vi "trash_Handle Late Iterations.vi"(8 "error in (no error)":errorcluster, 10 "Period (ns)":i64, 11 "CIFCorePlugin in":refnum<class "CIFCorePlugin.lvclass">) -> (0 "error out":errorcluster, 3 "CIFCorePlugin out":refnum<class "CIFCorePlugin.lvclass">)   [LabVIEW 2021, in "CIFCorePlugin.lvclass"]
uses:
  CIFCorePlugin.lvclass
  CIFCorePlugin.lvclass/CIFCorePlugin.ctl
  CIFUtilities/CIFClocks/Typedef/Errors.ctl
  Accessors/Read Iterations.vi
  Accessors/Get Time.vi
  Accessors/Timestamps/Read Running TS.vi
  CIFUtilities/CIFClocks/Core/Get Time.vi
  CIFUtilities/CIFClocks/Time Conversion/LabVIEW Time to UTC Time.vi
  CIFCoreCommon/CIFCoreCommon.lvlib
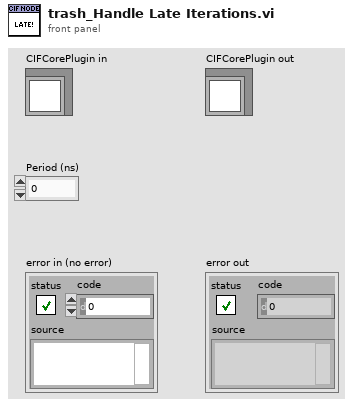
[diagram p1: front panel]
types:
  T1 = typedef "CIFCoreCommon.lvlib/Errors.ctl" = enum16{"Invalid Clock ID", "Long Sleep", "gRPC Server Not Found", "Config Parse", "Timestamp Wrap", "Delayed Execution"}
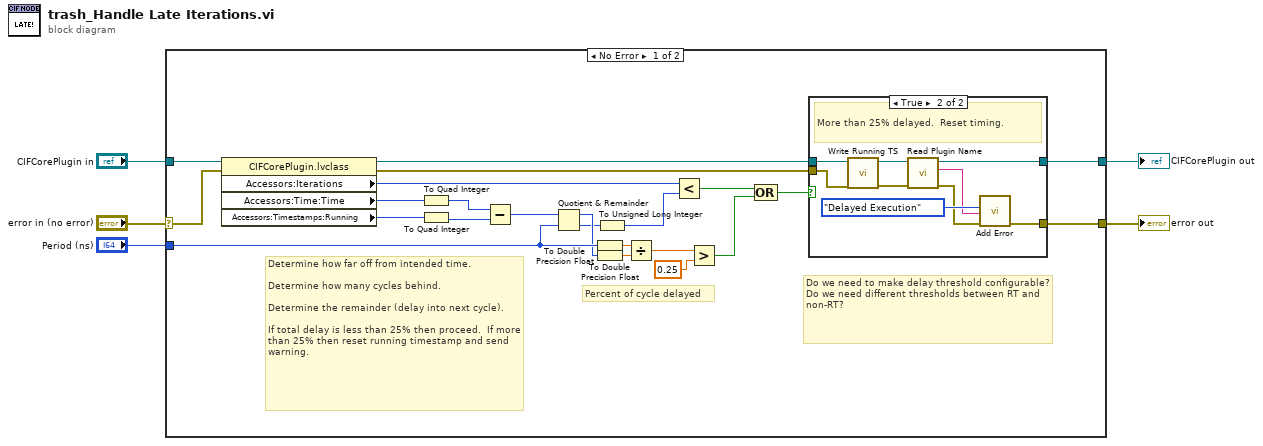
[diagram p0: block diagram]
diagram:
  n1 = case shown="No Error" "error in (no error)" {
    selector: "error in (no error)" -> [w8 w41]
    tunnel: [w7 w41] -> w4
    tunnel: [w10 w40] -> w2
    tunnel: "CIFCorePlugin in" -> [w28 w40]
    tunnel: "Period (ns)" -> [w22 _]
    frame No Error {
      # "Do we need to make delay threshold configurable?  Do we need different thresholds between RT and non-RT?"
      # "Determine how far off from intended time.\n\nDetermine how many cycles behind.\n\nDetermine the remainder (delay into next cycle).\n\nIf total delay is less than 25% then proceed.  If more than 25% then reset running timestamp and send warning."
      # "Percent of cycle delayed"
      n2 = property class="CIFCorePlugin.lvclass"(reference=w28, error in=w8) -> (reference out=w12:refnum<class "CIFCorePlugin.lvclass">, error out=w9:errorcluster, "Accessors:Iterations"=w15:u32, "Accessors:Time:Time"=w23:u64, "Accessors:Timestamps:Running"=w27:u64)
      n3 = To Quad Integer(1:w23) -> (0:w26:i64)
      n4 = To Quad Integer(1:w27) -> (0:w25:i64)
      n5 = Subtract(x=w26, y=w25) -> (x-y=w24:i64)
      n6 = Quotient & Remainder(x=w24, y=w22) -> (x-y*floor(x/y)=w21:i64, floor(x/y)=w16:i64)
      n7 = To Double Precision Float(number=w22) -> (double precision float=w19:dbl)
      n8 = To Double Precision Float(number=w21) -> (double precision float=w20:dbl)
      n9 = To Unsigned Long Integer(number=w16) -> (unsigned 32bit integer=w6:u32)
      n10 = Divide(x=w19, y=w20) -> (x/y=w18:dbl)
      n11 = Less?(x=w15, y=w6) -> (x < y?=w13:bool)
      n12 = Greater?(x=w18, y=0.25) -> (0:w14:bool)
      n13 = Compound Arithmetic op=OR(w13, w14) -> (w11:bool)
      n14 = case shown="True" w11 {
        tunnel: w12 -> [w30 w39]
        tunnel: [w30 w34] -> w10
        tunnel: w9 -> [w29 w38]
        tunnel: [w29 w33] -> w7
        frame False {
          # "Less and 25% of cycle delayed, keep running"
        }
        frame True {
          # "More than 25% delayed.  Reset timing."
          n15 = call "Write Running TS.vi"("error in (no error)"=w38, "CIFCorePlugin in"=w39) -> ("error out"=w31:errorcluster, "CIFCorePlugin out"=w32:refnum<class "CIFCorePlugin.lvclass">)  [unwired: 8 in]
          n16 = call "Read Plugin Name.vi"("error in (no error)"=w31, "CIFTemplateNode in"=w32) -> ("error out"=w35:errorcluster, "Plugin Name"=w36:string, "CIFTemplateNode out"=w34:refnum<class "CIFCorePlugin.lvclass">)  [unwired: 7 in]
          n17 = call "Add Error.vi"("error in (no error)"=w35, "String to Append"=w36, "Error"=Errors."Delayed Execution") -> ("error out"=w33:errorcluster)  [unwired: 8 in]
        }
      }
    }
    frame Error {
    }
  }
  "error out" <- w4
  "CIFCorePlugin out" <- w2
